vi "Model - Get Overhead.vi"(8 "error in (no error)":errorcluster, 11 "View Model":T6) -> (0 "error out":errorcluster, 2 "Overhead":T1={"Start"=FALSE, "Numeric"=0.0, "Blink CNTRLR1"=FALSE, "Blink CNTRLR2"=FALSE, "RT Status"={"Status TCL1"={"Duration, us"=0.0, "Late Counter"=0, "Timeout, us"=0}, "Status TCL2"={"Duration, us"=0.0, "Late Counter"=0, "Timeout, us"=0}, "Status NPL"={"Duration, us"=0.0, "Late Counter"=0, "Timeout, us"=0}, "Connected?"=FALSE}, "RT data"=[], "NStream"={"Endpoint"="", "exist?"=FALSE, "# elements"=125}, "Timer Data"={"ElapsedTime"=0.0, "Elapsed?"=FALSE, "Paused?"=FALSE}} {"RT Status"."Status NPL"."Duration, us" format="%0.2f"; "RT Status"."Status TCL2"."Duration, us" format="%0.2f"; "RT Status"."Status TCL1"."Duration, us" format="%0.2f"}, 3 "View Model":T6)   [LabVIEW 2017]
doc: "Get actual value of Controller Overhead from DVR"
uses:
  Controls/View Model.ctl
  Controls/Shared Model.ctl
  Error Handler/Controls/Error Model.ctl
  Error Handler/Controls/Error Event.ctl
  Error Handler/Controls/Error Type.ctl
  Controller/Controls/Controller Model.ctl
  Controller/Controls/Controller Event.ctl
  Controller/Controls/Controller Command.ctl
  Controller/Controls/Controller Overhead.ctl
  Real-Time/RT Status.ctl
  Real-Time/RT Loop Status.ctl
  Controller/Controls/Controller NStream.ctl
  Controller/Controls/Controller Timer Data.ctl
  Controller/Controls/Controller DAQ Data.ctl
  TDMS Logger/Controls/TDMS Model.ctl
  TDMS Logger/Controls/TDMS Event.ctl
  TDMS Logger/Controls/TDMS Command.ctl
  TDMS Logger/Controls/TDMS Overhead.ctl
  TDMS Logger/Controls/TDMS ChanProperties.ctl
  TDMS Logger/Controls/TDMS DAQ Data.ctl
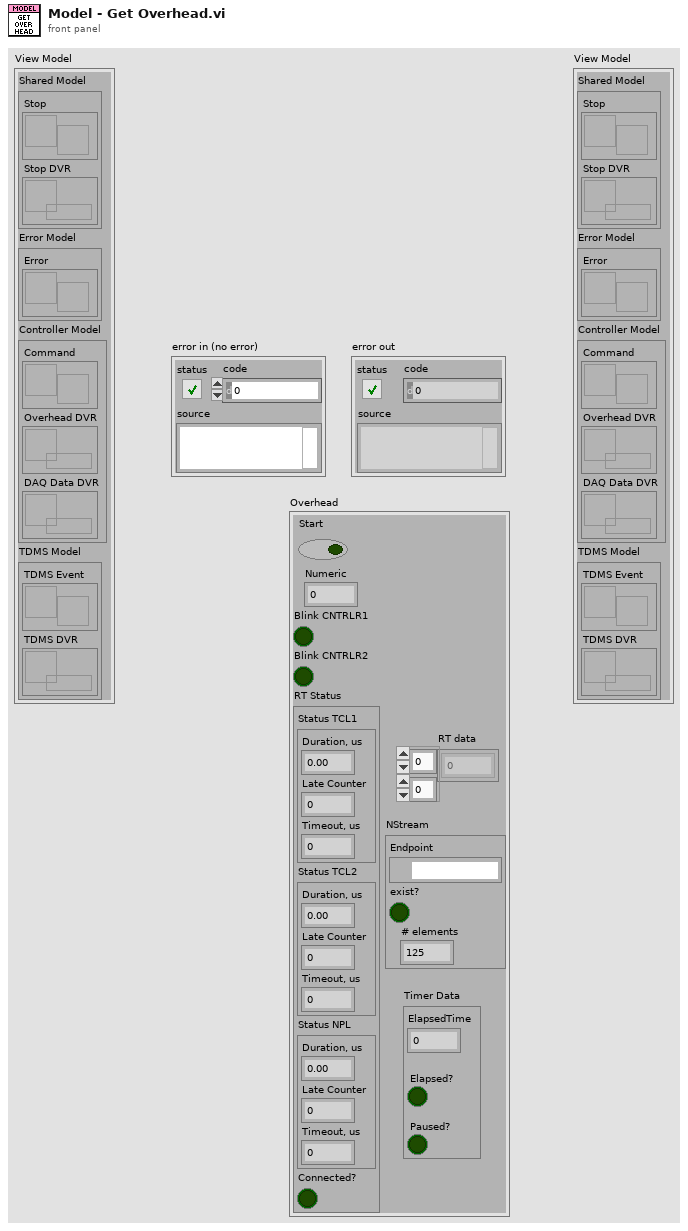
[diagram p1: front panel]
types:
  T1 = typedef "Controller Overhead.ctl" = cluster{"Start":bool, "Numeric":dbl, "Blink CNTRLR1":bool, "Blink CNTRLR2":bool, "RT Status":T2, "RT data":dbl[][], "NStream":T4, "Timer Data":T5}
  T2 = typedef "RT Status.ctl" = cluster{"Status TCL1":T3, "Status TCL2":T3, "Status NPL":T3, "Connected?":bool}
  T3 = typedef "RT Loop Status.ctl" = cluster{"Duration, us":dbl, "Late Counter":i32, "Timeout, us":u32}
  T4 = typedef "Controller NStream.ctl" = cluster{"Endpoint":refnum<k21>, "exist?":bool, "# elements":i32}
  T5 = typedef "Controller Timer Data.ctl" = cluster{"ElapsedTime":dbl, "Elapsed?":bool, "Paused?":bool}
  T6 = typedef "View Model.ctl" = cluster{"Shared Model":T7, "Error Model":T8, "Controller Model":T9, "TDMS Model":T10}
  T7 = typedef "Shared Model.ctl" = cluster{"Stop":refnum<user-event>, "Stop DVR":refnum<data-value>}
  T8 = typedef "Error Model.ctl" = cluster{"Error":refnum<user-event>}
  T9 = typedef "Controller Model.ctl" = cluster{"Command":refnum<user-event>, "Overhead DVR":refnum<data-value>, "DAQ Data DVR":refnum<data-value>}
  T10 = typedef "TDMS Model.ctl" = cluster{"TDMS Event":refnum<user-event>, "TDMS DVR":refnum<data-value>}
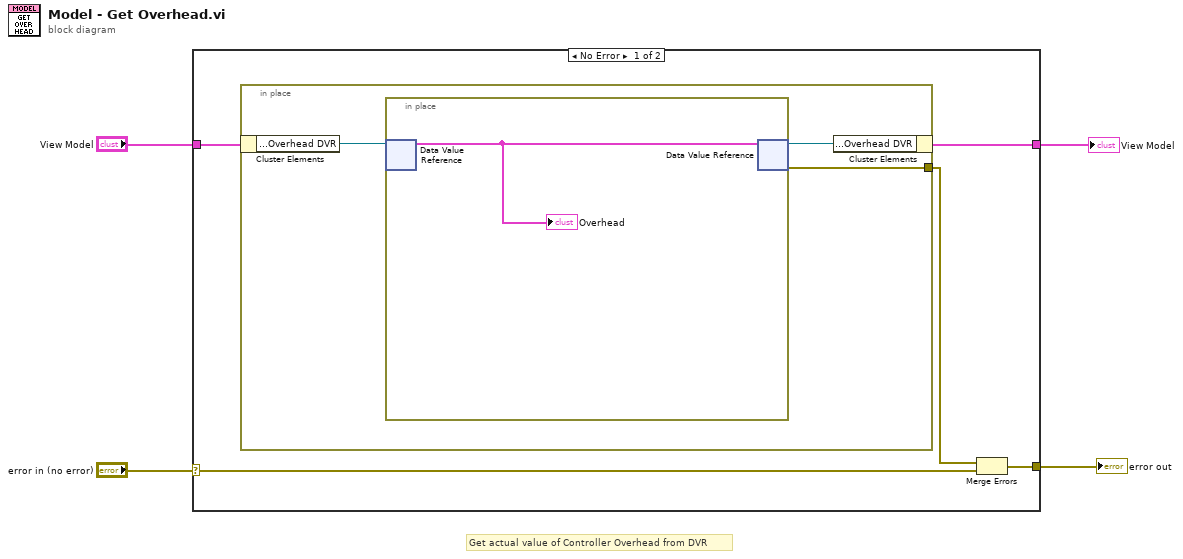
[diagram p0: block diagram]
diagram:
  # "Get actual value of Controller Overhead from DVR"
  n1 = case shown="No Error" "error in (no error)" {
    selector: "error in (no error)" -> [w6 w14]
    tunnel: "View Model" -> [w9 w15]
    tunnel: [w8 w15] -> w2
    tunnel: [w5 w14] -> w1
    frame No Error {
      n2 = in-place {
        in-place-border: [w10] -> w7
        n3 = in-place-cluster #1(w9) -> ("Controller Model.Overhead DVR"=w12:refnum<data-value>)
        n4 = in-place {
          n5 = in-place-dvr #2(w12) -> (w13:T1)  [unwired: 1 out]
          "Overhead" <- w13
          n6 = in-place-dvr #2(w13) -> (w11:refnum<data-value>, w10:errorcluster)
        }
        n7 = in-place-cluster #1("Controller Model.Overhead DVR"=w11) -> (w8:T6)
      }
      n8 = Merge Errors(w7, w6) -> (w5:errorcluster)
    }
    frame Error {
    }
  }
  "View Model" <- w2
  "error out" <- w1
